vi "Post Message.vi"(4 "Runtime Searching Path":path, 6 "Mode":enum32{"Devlopment", "Runtime"}(ring), 9 "Target Module":string, 10 "Arguments (\"\")":string, 11 "State":string) -> (0 "error out":errorcluster)   [LabVIEW 2020]
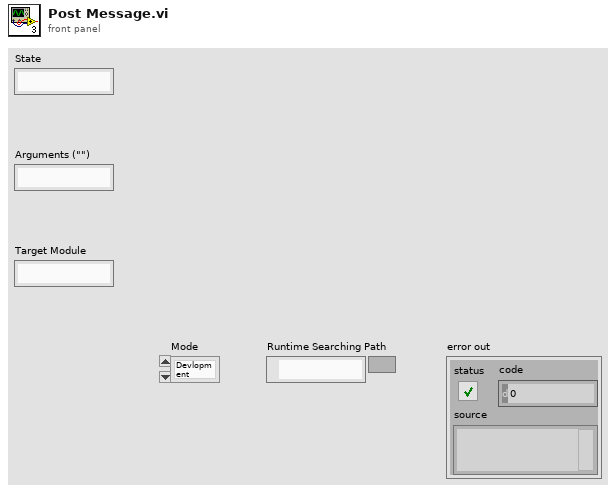
[diagram p1: front panel]
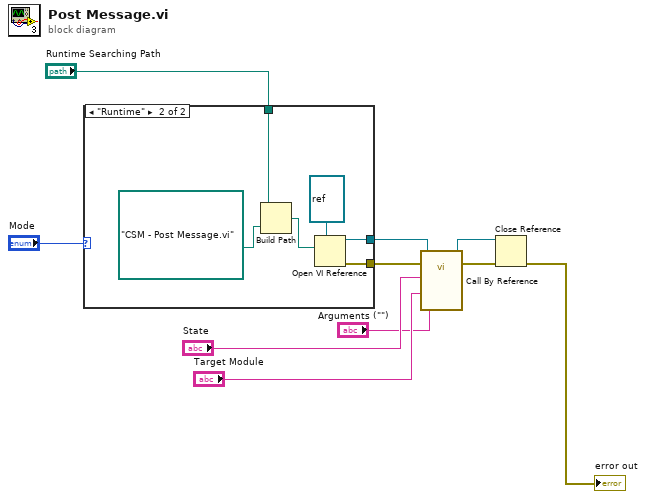
[diagram p0: block diagram]
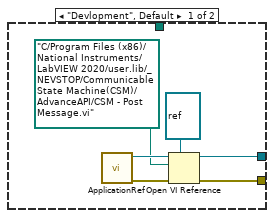
[diagram p2: hidden frame]
diagram:
  n1 = case shown="\"Runtime\"" "Mode" {
    tunnel: [w13 w21] -> w2
    tunnel: [w12 w20] -> w3
    tunnel: "Runtime Searching Path" -> [_ w17]
    frame "Devlopment", Default {
      n2 = call "ApplicationRef.vi"() -> ("error out"=w16:errorcluster, "Application out"=w15:refnum<vi>)  [unwired: 10 in]
      n3 = Open VI Reference(type specifier VI Refnum (for type only)=refnum<vi> refnum, application reference (local)=w15, vi path=path "C:/Program Files (x86)/National Instruments/LabVIEW 2020/user.lib/_NEVSTOP/Communicable State Machine(CSM)/AdvanceAPI/CSM - Post Message.vi", error in (no error)=w16) -> (vi reference=w12:refnum<vi>, error out=w13:errorcluster)  [unwired: 2 in]
    }
    frame "Runtime" {
      n4 = Build Path(base path=w17, name or relative path=path "CSM - Post Message.vi" ("vi path")) -> (appended path=w18:path)
      n5 = Open VI Reference(type specifier VI Refnum (for type only)=refnum<vi> refnum, vi path=w18) -> (vi reference=w20:refnum<vi>, error out=w21:errorcluster)  [unwired: 4 in]
    }
  }
  n6 = call-by-ref "?"(reference=w3, error in=w2, "Target Module"="Target Module", "Arguments (\"\")"="Arguments (\"\")", "State"="State") -> (reference out=w5:refnum<vi>, error out=w4:errorcluster)  [unwired: 8 in, 1 out]
  n7 = Close Reference(reference=w5, error in (no error)=w4) -> (error out=→"error out":errorcluster)
